vi "AIM 664 test Import Configuration File (Non Default Attributes).vi"(8 "error in (no error)":errorcluster, 11 "TestCase in":refnum<class "AIM 664 Import.lvclass">) -> (0 "error out":errorcluster, 3 "TestCase out":refnum<class "AIM 664 Import.lvclass">)   [LabVIEW 2020, in "AIM 664 Import.lvclass"]
uses:
  AIM 664 Import.lvclass
  Shared/Port Session Configuration.ctl
  Shared/board_setup.ctl
  Shared/port_configuration.ctl
  Shared/port_setup.ctl
  Shared/tx_udp_setup.ctl
  Shared/port_tx_udp_comm.ctl
  Shared/frame_parameter.ctl
  Shared/frame_parameter_definition.ctl
  <vilib>/NI/NI VeriStand Encoding and Decoding/Encoding.ctl
  Shared/port_tx_udp_sap.ctl
  Shared/rx_udp_setup.ctl
  Shared/port_rx_udp_comm.ctl
  Shared/port_rx_udp_sap.ctl
  <vilib>/addons/_JKI Toolkits/VI Tester/TestCase.llb/TestCase.lvclass
  <vilib>/NI/VeriStand Custom Device Testing Tools/VeriStandTestUtilities/VeriStandTestUtilities.lvlib
  Import/AIM ARINC 664 Import.lvlib
  <vilib>/NI/NI VeriStand Encoding and Decoding/Encoding and Decoding.lvlib
  C:/Program Files (x86)/National Instruments/LabVIEW 2020/vi.lib/addons/_JKI Toolkits/VI Tester/TestCase.llb/TestCase.lvclass
panel:
  out "x = y? 2":bool[](array[boolean])
  out "logical AND 6":bool
  out "index of element":i32[](array[numeric])
  out "size(s)":i32
  out "x = y?":T1
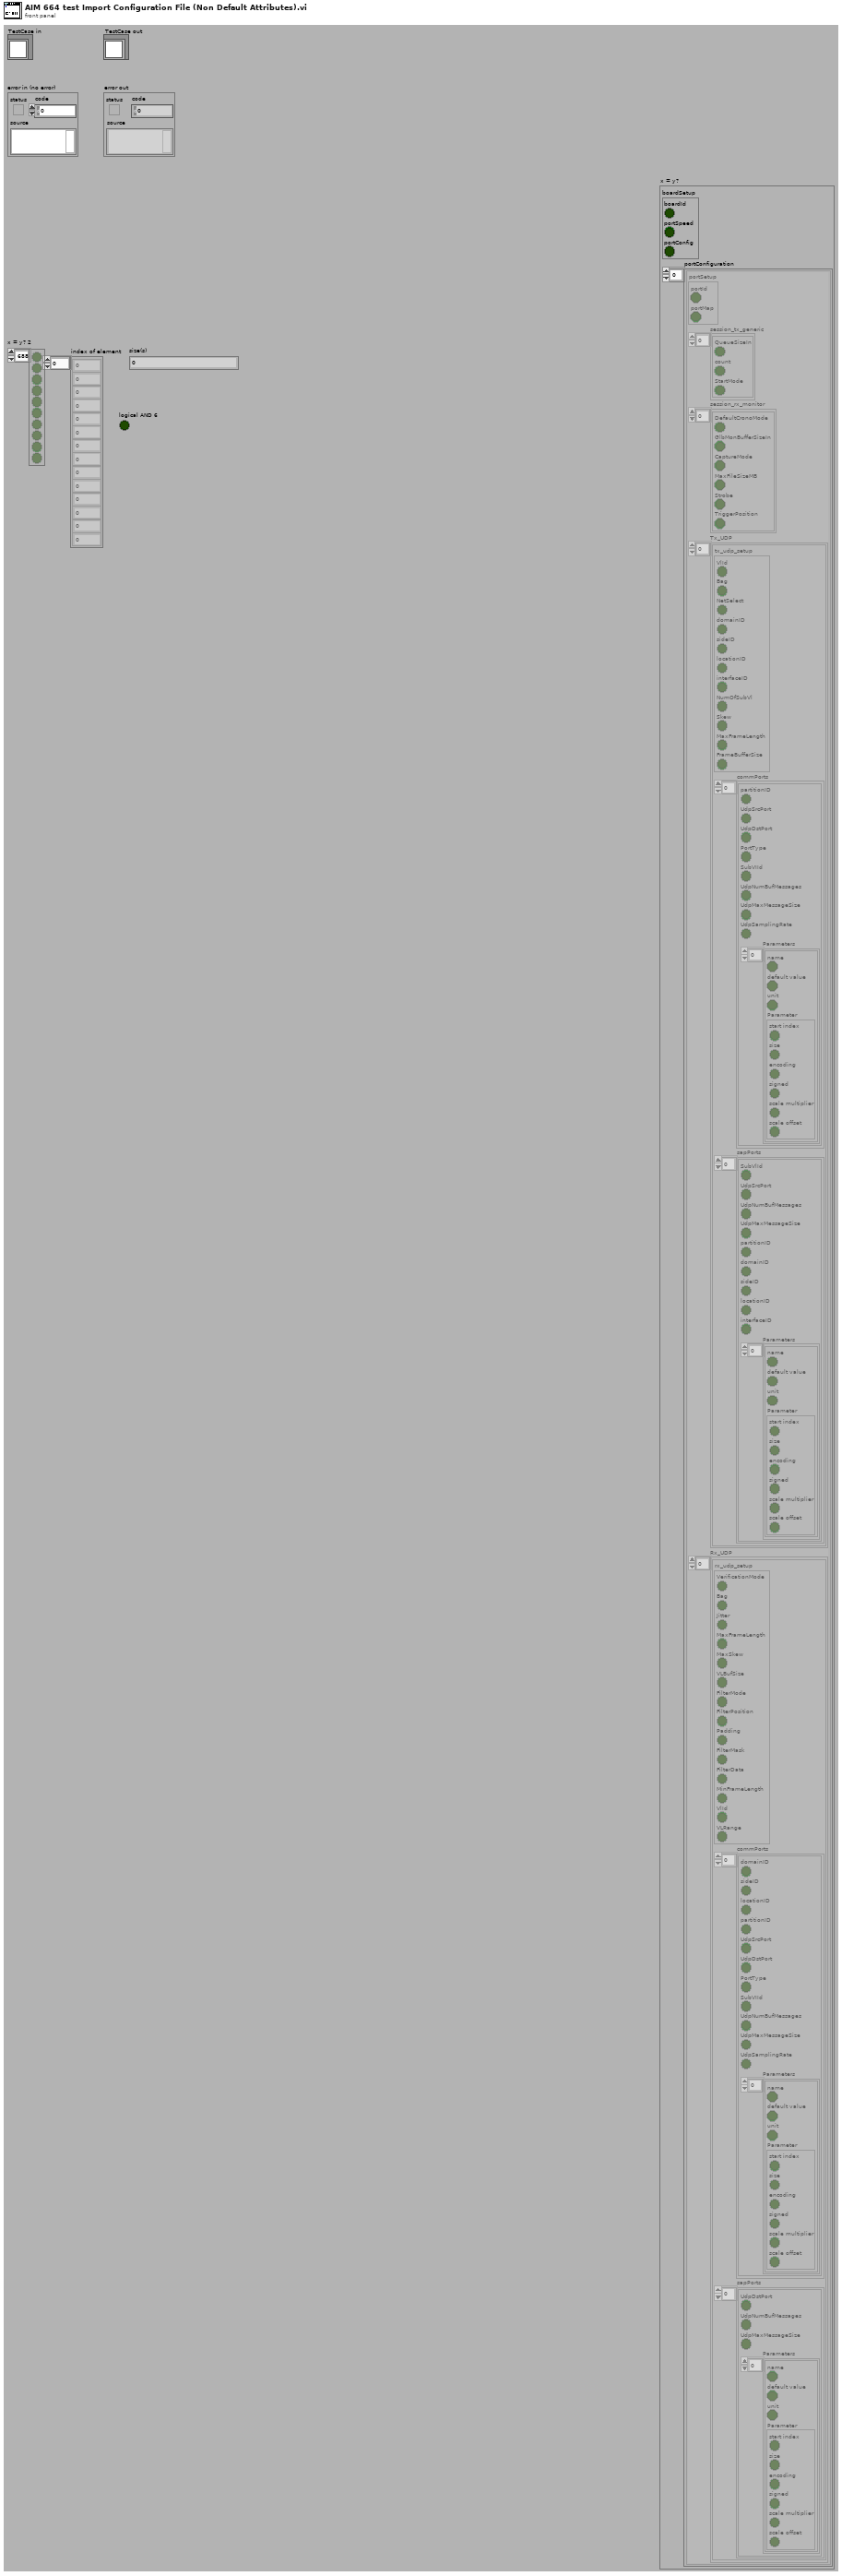
[diagram p1: front panel]
types:
  T1 = cluster{"boardSetup":cluster{"boardId":bool, "portSpeed":bool, "portConfig":bool}, "portConfiguration":cluster{"portSetup":cluster{"portId":bool, "portMap":bool}, "session_tx_generic":cluster{"QueueSizeIn":bool, "count":bool, "StartMode":bool}[], "session_rx_monitor":cluster{"DefaultCronoMode":bool, "GlbMonBufferSizeIn":bool, "CaptureMode":bool, "MaxFileSizeMB":bool, "Strobe":bool, "TriggerPosition":bool}[], "Tx_UDP":cluster{"tx_udp_setup":cluster{"VlId":bool, "Bag":bool, "NetSelect":bool, "domainID":bool, "sideID":bool, "locationID":bool, "interfaceID":bool, "NumOfSubVl":bool, "Skew":bool, "MaxFrameLength":bool, "FrameBufferSize":bool}, "commPorts":cluster{"partitionID":bool, "UdpSrcPort":bool, "UdpDstPort":bool, "PortType":bool, "SubVIId":bool, "UdpNumBufMessages":bool, "UdpMaxMessageSize":bool, "UdpSamplingRate":bool, "Parameters":cluster{"name":bool, "default value":bool, "unit":bool, "Parameter":cluster{"start index":bool, "size":bool, "encoding":bool, "signed":bool, "scale multiplier":bool, "scale offset":bool}}[]}[], "sapPorts":cluster{"SubVlId":bool, "UdpSrcPort":bool, "UdpNumBufMessages":bool, "UdpMaxMessageSize":bool, "partitionID":bool, "domainID":bool, "sideID":bool, "locationID":bool, "interfaceID":bool, "Parameters":cluster{"name":bool, "default value":bool, "unit":bool, "Parameter":cluster{"start index":bool, "size":bool, "encoding":bool, "signed":bool, "scale multiplier":bool, "scale offset":bool}}[]}[]}[], "Rx_UDP":cluster{"rx_udp_setup":cluster{"VerificationMode":bool, "Bag":bool, "Jitter":bool, "MaxFrameLength":bool, "MaxSkew":bool, "VLBufSize":bool, "FilterMode":bool, "FilterPosition":bool, "Padding":bool, "FilterMask":bool, "FilterData":bool, "MinFrameLength":bool, "VlId":bool, "VLRange":bool}, "commPorts":cluster{"domainID":bool, "sideID":bool, "locationID":bool, "partitionID":bool, "UdpSrcPort":bool, "UdpDstPort":bool, "PortType":bool, "SubVIId":bool, "UdpNumBufMessages":bool, "UdpMaxMessageSize":bool, "UdpSamplingRate":bool, "Parameters":cluster{"name":bool, "default value":bool, "unit":bool, "Parameter":cluster{"start index":bool, "size":bool, "encoding":bool, "signed":bool, "scale multiplier":bool, "scale offset":bool}}[]}[], "sapPorts":cluster{"UdpDstPort":bool, "UdpNumBufMessages":bool, "UdpMaxMessageSize":bool, "Parameters":cluster{"name":bool, "default value":bool, "unit":bool, "Parameter":cluster{"start index":bool, "size":bool, "encoding":bool, "signed":bool, "scale multiplier":bool, "scale offset":bool}}[]}[]}[]}[]}
  T2 = typedef "AIM ARINC 664 Import.lvlib/Port Session Configuration.ctl" = cluster{"boardSetup":T3, "portConfiguration":T4[]}
  T3 = typedef "AIM ARINC 664 Import.lvlib/board_setup.ctl" = cluster{"boardId":u32, "portSpeed":u32, "portConfig":u32}
  T4 = typedef "AIM ARINC 664 Import.lvlib/port_configuration.ctl" = cluster{"portSetup":T5, "session_tx_generic":cluster{"QueueSizeIn":u32, "count":i32, "StartMode":i32}[], "session_rx_monitor":cluster{"DefaultCronoMode":u32, "GlbMonBufferSizeIn":u32, "CaptureMode":u32, "MaxFileSizeMB":u32, "Strobe":u32, "TriggerPosition":u32}[], "Tx_UDP":cluster{"tx_udp_setup":T6, "commPorts":T7[], "sapPorts":T11[]}[], "Rx_UDP":cluster{"rx_udp_setup":T12, "commPorts":T13[], "sapPorts":T14[]}[]}
  T5 = typedef "AIM ARINC 664 Import.lvlib/port_setup.ctl" = cluster{"portId":u32, "portMap":u32}
  T6 = typedef "AIM ARINC 664 Import.lvlib/tx_udp_setup.ctl" = cluster{"VlId":i32, "Bag":i32, "NetSelect":i32, "domainID":u8, "sideID":u8, "locationID":u8, "interfaceID":u8, "NumOfSubVl":u16, "Skew":u32, "MaxFrameLength":u32, "FrameBufferSize":u32}
  T7 = typedef "AIM ARINC 664 Import.lvlib/port_tx_udp_comm.ctl" = cluster{"partitionID":u8, "UdpSrcPort":u16, "UdpDstPort":u16, "PortType":enum16{"FDX_UDP_SAMPLING", "FDX_UDP_QUEUING"}, "SubVIId":u32, "UdpNumBufMessages":u32, "UdpMaxMessageSize":u32, "UdpSamplingRate":u32, "Parameters":T8[]}
  T8 = typedef "AIM ARINC 664 Import.lvlib/frame_parameter.ctl" = cluster{"name":string, "default value":dbl, "unit":string, "Parameter":T9}
  T9 = typedef "AIM ARINC 664 Import.lvlib/frame_parameter_definition.ctl" = cluster{"start index":i32, "size":i32, "encoding":T10, "signed":bool, "scale multiplier":dbl, "scale offset":dbl}
  T10 = typedef "Encoding and Decoding.lvlib/Encoding.ctl" = enum16{"BNR", "BCD", "Discrete"}
  T11 = typedef "AIM ARINC 664 Import.lvlib/port_tx_udp_sap.ctl" = cluster{"SubVlId":u8, "UdpSrcPort":u16, "UdpNumBufMessages":u32, "UdpMaxMessageSize":u32, "partitionID":u8, "domainID":u8, "sideID":u8, "locationID":u8, "interfaceID":u8, "Parameters":T8[]}
  T12 = typedef "AIM ARINC 664 Import.lvlib/rx_udp_setup.ctl" = cluster{"VerificationMode":u32, "Bag":u32, "Jitter":u32, "MaxFrameLength":u32, "MaxSkew":u32, "VLBufSize":u32, "FilterMode":u32, "FilterPosition":u32, "Padding":u32, "FilterMask":u32, "FilterData":u32, "MinFrameLength":u32, "VlId":u16, "VLRange":u32}
  T13 = typedef "AIM ARINC 664 Import.lvlib/port_rx_udp_comm.ctl" = cluster{"domainID":u8, "sideID":u8, "locationID":u8, "partitionID":u8, "UdpSrcPort":u16, "UdpDstPort":u16, "PortType":enum16{"FDX_UDP_SAMPLING", "FDX_UDP_QUEUING"}, "SubVIId":u32, "UdpNumBufMessages":u32, "UdpMaxMessageSize":u32, "UdpSamplingRate":u32, "Parameters":T8[]}
  T14 = typedef "AIM ARINC 664 Import.lvlib/port_rx_udp_sap.ctl" = cluster{"UdpDstPort":u16, "UdpNumBufMessages":u32, "UdpMaxMessageSize":u32, "Parameters":T8[]}
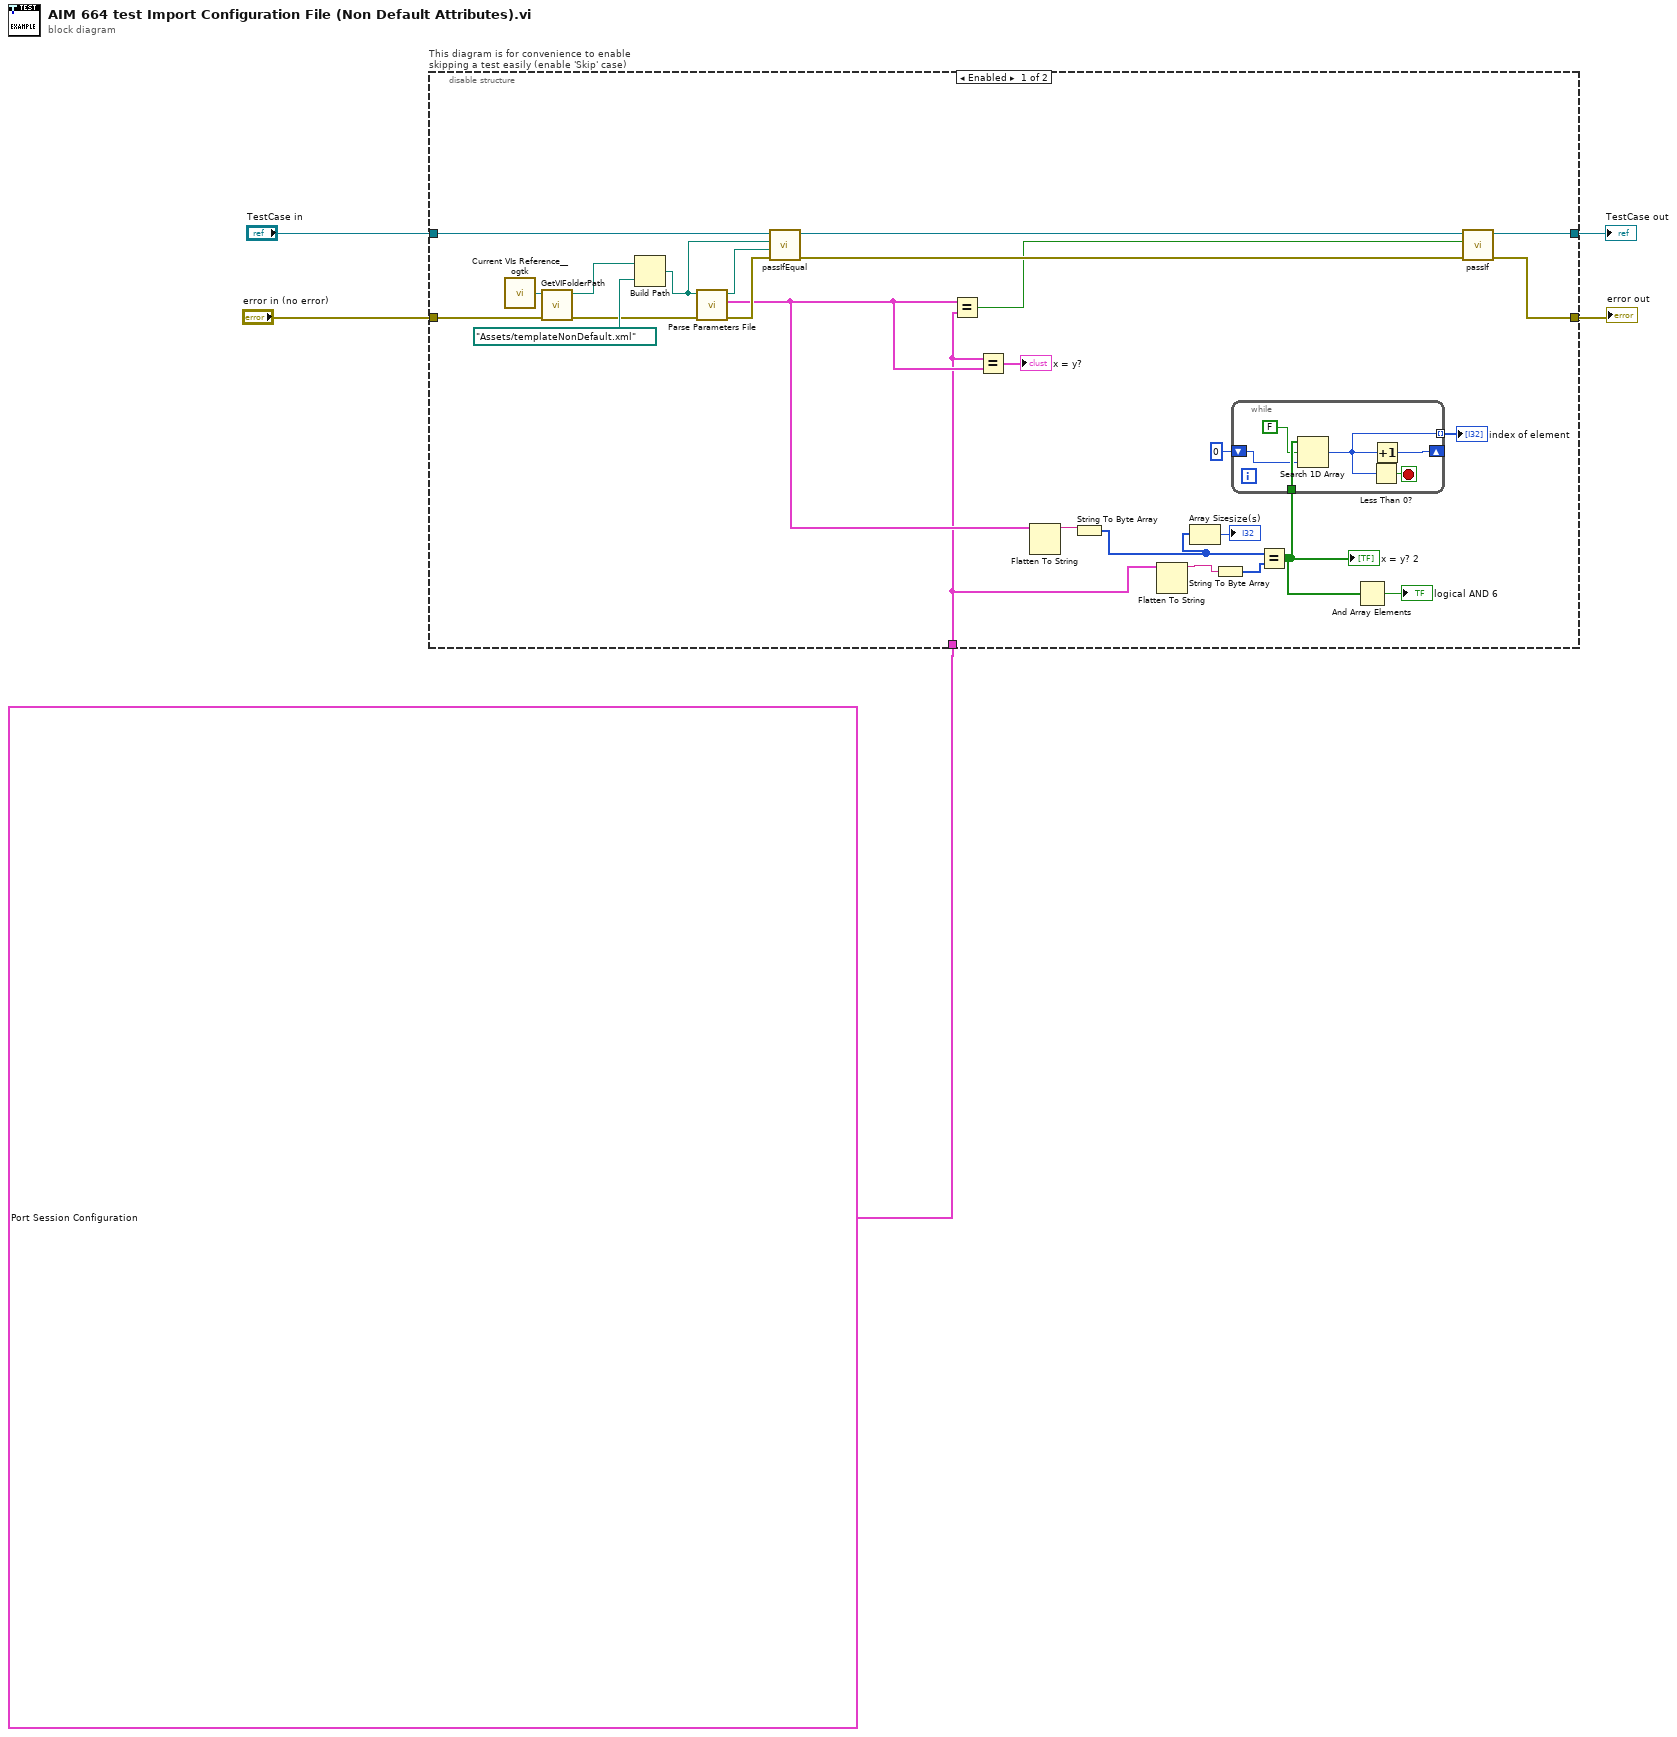
[diagram p0: block diagram]
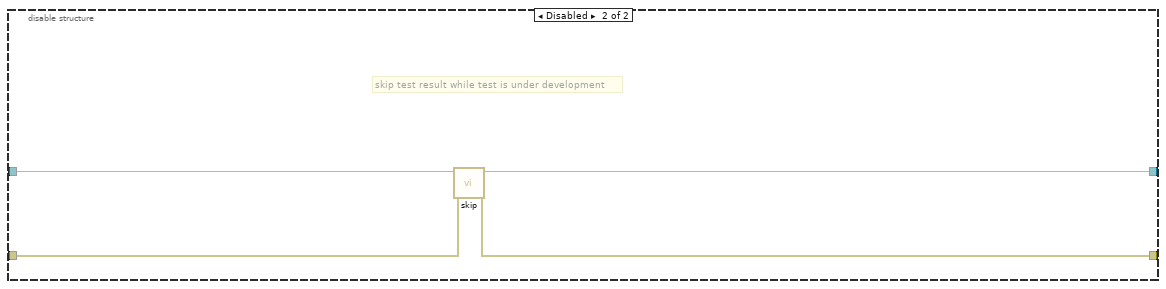
[diagram p2: hidden frame]
diagram:
  n1 = disable-structure "This diagram is for convenience to enable skipping a test easily (enable 'Skip' case)" shown="Enabled" {
    disable-tunnel: "TestCase in" -> [w24 w41]
    disable-tunnel: [w26 w39] -> w2
    disable-tunnel: [w25 w40] -> w4
    disable-tunnel: "error in (no error)" -> [w29 w38]
    disable-tunnel: T2 {"boardSetup"={"boardId"=1, "portSpeed"=1, "portConfig"=1}, "portConfiguration"=[{"portSetup"={"portId"=2, "portMap"=1}, "session_tx_generic"=[{"QueueSizeIn"=3, "count"=6, "StartMode"=3}], "session_rx_monitor"=[{"DefaultCronoMode"=2, "GlbMonBufferSizeIn"=2, "CaptureMode"=3, "MaxFileSizeMB"=4, "Strobe"=2, "TriggerPosition"=3}], "Tx_UDP"=[], "Rx_UDP"=[]}, {"portSetup"={"portId"=3, "portMap"=2}, "session_tx_generic"=[], "session_rx_monitor"=[], "Tx_UDP"=[{"tx_udp_setup"={"VlId"=4, "Bag"=2, "NetSelect"=3, "domainID"=1, "sideID"=12, "locationID"=2, "interfaceID"=2, "NumOfSubVl"=3, "Skew"=5, "MaxFrameLength"=3, "FrameBufferSize"=1}, "commPorts"=[{"partitionID"=123, "UdpSrcPort"=444, "UdpDstPort"=22, "PortType"=enum."FDX_UDP_QUEUING", "SubVIId"=233, "UdpNumBufMessages"=2425, "UdpMaxMessageSize"=11, "UdpSamplingRate"=344, "Parameters"=[{"name"="Param 0", "default value"=1.0, "unit"="x", "Parameter"={"start index"=2, "size"=29, "encoding"=enum."BCD", "signed"=TRUE, "scale multiplier"=3.14, "scale offset"=2.0}}, {"name"="Param 1", "default value"=1.0, "unit"="x", "Parameter"={"start index"=2, "size"=29, "encoding"=enum."BCD", "signed"=TRUE, "scale multiplier"=3.14, "scale offset"=2.0}}, {"name"="Param 2", "default value"=1.0, "unit"="x", "Parameter"={"start index"=2, "size"=29, "encoding"=enum."BCD", "signed"=TRUE, "scale multiplier"=3.14, "scale offset"=2.0}}]}], "sapPorts"=[{"SubVlId"=4, "UdpSrcPort"=123, "UdpNumBufMessages"=134, "UdpMaxMessageSize"=4, "partitionID"=6, "domainID"=2, "sideID"=8, "locationID"=5, "interfaceID"=4, "Parameters"=[{"name"="Param 0", "default value"=1.0, "unit"="x", "Parameter"={"start index"=2, "size"=29, "encoding"=enum."BCD", "signed"=TRUE, "scale multiplier"=3.14, "scale offset"=2.0}}, {"name"="Param 1", "default value"=1.0, "unit"="x", "Parameter"={"start index"=2, "size"=29, "encoding"=enum."BCD", "signed"=TRUE, "scale multiplier"=3.14, "scale offset"=2.0}}, {"name"="Param 2", "default value"=1.0, "unit"="x", "Parameter"={"start index"=2, "size"=29, "encoding"=enum."BCD", "signed"=TRUE, "scale multiplier"=3.14, "scale offset"=2.0}}]}]}], "Rx_UDP"=[{"rx_udp_setup"={"VerificationMode"=4, "Bag"=2, "Jitter"=2, "MaxFrameLength"=8, "MaxSkew"=6, "VLBufSize"=44, "FilterMode"=1, "FilterPosition"=5, "Padding"=0, "FilterMask"=6, "FilterData"=4, "MinFrameLength"=46, "VlId"=34, "VLRange"=33}, "commPorts"=[{"domainID"=1, "sideID"=4, "locationID"=3, "partitionID"=4, "UdpSrcPort"=245, "UdpDstPort"=4, "PortType"=enum."FDX_UDP_QUEUING", "SubVIId"=0, "UdpNumBufMessages"=8, "UdpMaxMessageSize"=6, "UdpSamplingRate"=0, "Parameters"=[{"name"="Param 0", "default value"=0.0, "unit"="", "Parameter"={"start index"=0, "size"=0, "encoding"=enum."BNR", "signed"=FALSE, "scale multiplier"=0.0, "scale offset"=0.0}}, {"name"="Param 1", "default value"=0.0, "unit"="", "Parameter"={"start index"=0, "size"=0, "encoding"=enum."BNR", "signed"=FALSE, "scale multiplier"=0.0, "scale offset"=0.0}}]}], "sapPorts"=[{"UdpDstPort"=1, "UdpNumBufMessages"=3, "UdpMaxMessageSize"=2, "Parameters"=[{"name"="Param 0", "default value"=0.0, "unit"="", "Parameter"={"start index"=0, "size"=0, "encoding"=enum."BNR", "signed"=FALSE, "scale multiplier"=0.0, "scale offset"=0.0}}, {"name"="Param 1", "default value"=0.0, "unit"="", "Parameter"={"start index"=0, "size"=0, "encoding"=enum."BNR", "signed"=FALSE, "scale multiplier"=0.0, "scale offset"=0.0}}]}]}]}]} ("board configuration") -> [w6 _]
    frame Enabled {
      n2 = call <userlib>:"Current VIs Reference__ogtk.vi"() -> ("Current VI's reference"=w31:refnum<vi>)  [unwired: 5 in]
      n3 = call <vilib>:"GetVIFolderPath.vi"("error in (no error)"=w29, "VI Reference in"=w31) -> ("error out"=w27:errorcluster, "VI Folder Path out"=w30:path)  [unwired: 8 in]
      n4 = Build Path(base path=w30, name or relative path=path "Assets/templateNonDefault.xml") -> (appended path=w21:path)
      n5 = call "Parse Parameters File.vi"("error in"=w27, "path to XML document"=w21) -> ("error out"=w22:errorcluster, "board configuration"=w7:T2, "path to XML document out"=w20:path)  [unwired: 7 in]
      n6 = call-dynamic "passIfEqual.vi"("error in (no error)"=w22, "y"=w20, "x"=w21, "TestCase in"=w24) -> ("error out"=w19:errorcluster, "TestCase out"=w23:refnum<class "AIM 664 Import.lvclass">)  [unwired: 6 in]
      n7 = Equal?(x=w7, y=w6) -> (x = y?=w18:bool)
      n8 = Equal?(x=w6, y=w7) -> (x = y?=→"x = y?":T1)
      n9 = Flatten To String(anything=w7) -> (data string=w16:string)  [unwired: 3 in, 2 out]
      n10 = String To Byte Array(string=w16) -> (unsigned byte array=w11:u8[])
      n11 = Flatten To String(anything=w6) -> (data string=w15:string)  [unwired: 3 in, 2 out]
      n12 = Array Size(array=w11) -> (size(s)=→"size(s)":i32)
      n13 = String To Byte Array(string=w15) -> (unsigned byte array=w14:u8[])
      n14 = Equal?(x=w11, y=w14) -> (x = y?=w12:bool[])
      "x = y? 2" <- w12
      n15 = while {
        tunnel: w12 -> [w37]
        tunnel: [w34] -> w9 mode=indexing
        shift-right: [w32] -> _
        shift-left: 0 ("index of element") -> [w33]
        stop <- w35 stop-if-true
        n16 = Search 1D Array(1D array=w37, element=FALSE ("logical AND 6"), start index (0)=w33) -> (index of element=w34:i32)
        n17 = Less Than 0?(x=w34) -> (x < 0?=w35:bool)
        n18 = Increment(x=w34) -> (x+1=w32:i32)
      }
      "index of element" <- w9
      n19 = And Array Elements(Boolean array=w12) -> (logical AND=→"logical AND 6":bool)
      n20 = call-dynamic "passIf.vi"("error in (no error)"=w19, "pass"=w18, "TestCase in"=w23) -> ("error out"=w25:errorcluster, "TestCase out"=w26:refnum<class "AIM 664 Import.lvclass">)  [unwired: 7 in]
    }
    frame Disabled {
      # "skip test result while test is under development"
      n21 = call <vilib>:"skip.vi"("error in (no error)"=w38, "TestCase in"=w41) -> ("error out"=w40:errorcluster, "TestCase out"=w39:refnum<class "AIM 664 Import.lvclass">)  [unwired: 8 in]
    }
  }
  "error out" <- w4
  "TestCase out" <- w2
